vi "SetExposure.vi"(8 "error in (no error)":errorcluster, 10 "Exposure(ms)":dbl, 11 "Hamamatsu_Camera in":refnum<class "Hamamatsu_Camera.lvclass">) -> (0 "error out":errorcluster, 3 "Hamamatsu_Camera out":refnum<class "Hamamatsu_Camera.lvclass">)   [LabVIEW 2023, in "CameraLibrary.lvlib" / "Hamamatsu_Camera.lvlib" / "Hamamatsu_Camera.lvclass"]
uses:
  Hamamatsu_Camera.lvclass
  Hamamatsu_Camera.lvclass/Hamamatsu_Camera.ctl
  Interfaces/AbstractInstrumentClasses/Cameras_LV/CameraComm Messages/Exposure Set Msg/Exposure Set Msg.lvclass
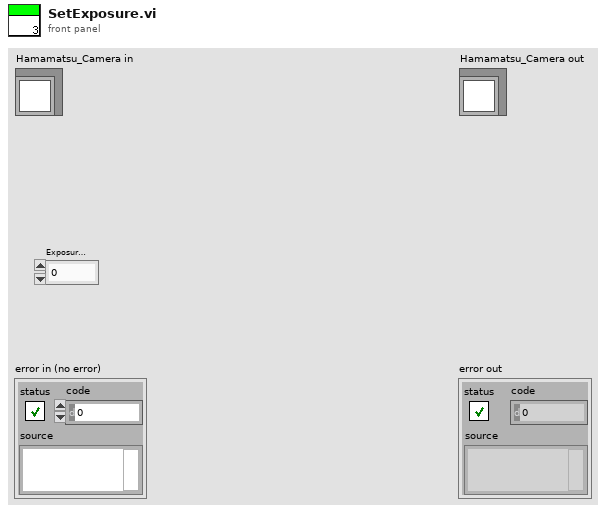
[diagram p1: front panel]
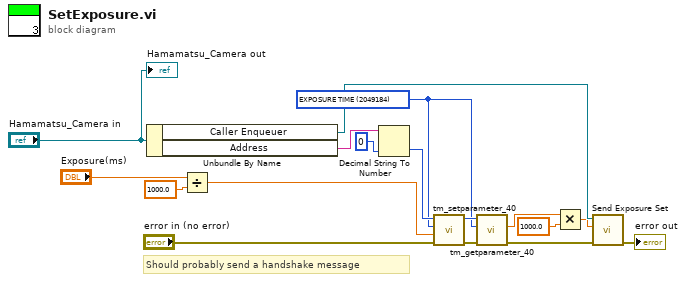
[diagram p0: block diagram]
diagram:
  w4 = u32 2049184 items=["SENSOR MODE"=4212128, "SENSOR MODE LINE BUNDLE HEIGHT"=4212192, "READOUT DIRECTION"=4211904, "BIT PER CHANNEL"=4342976, "EXPOSURE TIME"=2049184, "CONTRAST GAIN"=3163312, "BINNING"=4215968, "TIMING READOUT TIME"=4223904, "INTERNAL FRAME RATE"=4225952, "INTERNAL FRAME INTERVAL"=4225968, "INTERNAL LINE SPEED"=4226000, "IMAGE WIDTH"=4343200, "IMAGE HEIGHT"=4343216, "IMAGE ROWBYTES"=4343232, "IMAGE FRAMEBYTES"=4343248, "IMAGE PIXEL TYPE"=4343296] ("Parameter")
  # "Should probably send a handshake message"
  n1 = Unbundle By Name("Hamamatsu_Camera in") -> ("Caller Enqueuer"=w9:refnum<class "Message Enqueuer.lvclass">, "Address"=w15:string)
  n2 = Divide(x="Exposure(ms)", y=1000.0) -> (x/y=w10:dbl)
  n3 = Decimal String To Number(string=w15, default (0L)=u32 0 ("default (0 I32)")) -> (number=w14:u32)  [unwired: 1 in, 1 out]
  n4 = call "tm_setparameter_40.vi"("error in (no error)"="error in (no error)", "Value in"=w10, "Parameter"=w4, "Handle in"=w14) -> ("error out"=w6:errorcluster, "Handle out"=w7:u32)  [unwired: 6 in]
  n5 = call "tm_getparameter_40.vi"("error in (no error)"=w6, "Parameter"=w4, "Handle in"=w7) -> ("error out"=w5:errorcluster, "Value out"=w2:dbl)  [unwired: 6 in, 1 out]
  n6 = Multiply(x=w2, y=1000.0) -> (x*y=w1:dbl)
  n7 = call "Send Exposure Set.vi"("error in (no error)"=w5, "Exposure(ms)"=w1, "Message Enqueuer"=w9) -> ("error out"=→"error out":errorcluster)  [unwired: 7 in, 1 out]
  "Hamamatsu_Camera out" <- "Hamamatsu_Camera in"
